vi "Channels to Display Strings and Indices.vi"(9 "Instance ID":string, 10 "Channels":refnum<class "TBM channel.lvclass">[](array[class]), 11 "engine configuration in":refnum<class "engine configuration.lvclass">) -> (3 "display strings and indices":T1(array[cluster]))   [LabVIEW 2014, in "GraphViz Mapping Visualizer.lvlib"]
uses:
  GraphViz Mapping Visualizer.lvlib
  <vilib>/NI/Tag Bus Module Framework/channel/TBM channel.lvclass
  <vilib>/NI/Module Execution Interface/Engine Configuration/engine configuration.lvclass
  <vilib>/NI/Tag Bus/tag/tag descriptor.lvclass/tag descriptor.ctl
  <vilib>/NI/Tag Bus/tag/read tag name.vi
  <vilib>/NI/Tag Bus/tag/tag descriptor.lvclass
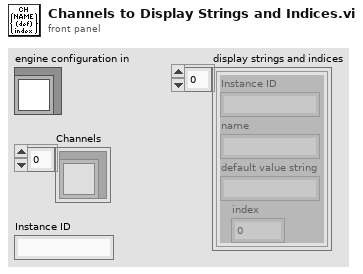
[diagram p1: front panel]
types:
  T1 = cluster{"Instance ID":string, "name":string, "default value string":string, "index":i32}[]
  T2 = cluster{"Instance ID":string, "name":string, "default value string":string, "index":i32}
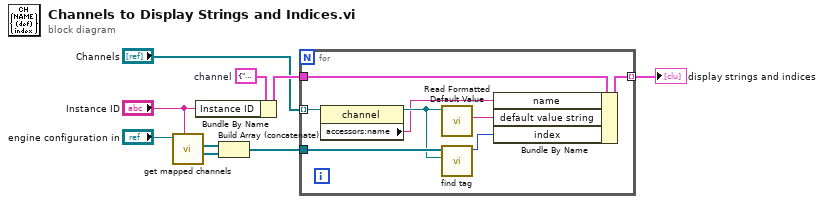
[diagram p0: block diagram]
diagram:
  w6 = T2 {"Instance ID"="", "name"="", "default value string"="", "index"=0}  # channel
  n1 = call-dynamic "get mapped channels.vi"("owner"="Instance ID", "engine configuration in"="engine configuration in") -> ("write channels"=w3:refnum<class "TBM channel.lvclass">[], "read channels"=w2:refnum<class "TBM channel.lvclass">[])  [unwired: 5 in, 3 out]
  n2 = Bundle By Name(cluster=w6, "Instance ID"="Instance ID") -> (w7:T2)
  n3 = Build Array (concatenate)(w2, w3) -> (w5:refnum<class "TBM channel.lvclass">[])
  n4 = for {
    tunnel: "Channels" -> [w17] mode=indexing
    tunnel: w5 -> [w16]
    tunnel: [w11] -> w9 mode=indexing
    tunnel: w7 -> [w10]
    n5 = property class="channel"(reference=w17) -> (reference out=w15:refnum<class "TBM channel.lvclass">, "accessors:name"=w14:string)  [unwired: 1 in, 1 out]
    n6 = call "Read Formatted Default Value.vi"("channel"=w15) -> ("Formatted Default"=w13:string)  [unwired: 9 in, 1 out]
    n7 = call <vilib>:"find tag.vi"("tag"=w15, "tags in"=w16) -> ("index"=w12:i32)  [unwired: 9 in]
    n8 = Bundle By Name(cluster=w10, "name"=w14, "default value string"=w13, "index"=w12) -> (w11:T2)
  }
  "display strings and indices" <- w9
